vi "Initialize Actor.vi"(7 "Host Name":string, 8 "error in (no error)":errorcluster, 9 "Actor Name":string, 10 "Message Broker Interface":refnum<class "Message Broker Interface.lvclass">, 11 "WS Server in":refnum<class "WS Server.lvclass">) -> (0 "error out":errorcluster, 3 "WS Server out":refnum<class "WS Server.lvclass">)   [LabVIEW 2016, in "WebSocket Networking.lvlib" / "WS Server.lvclass"]
doc: "--\nCopyright © 2017 Composed SystemsI All rights reserved.\n\nAuthor: Jon McBee <jon.mcbee@composed.io>\n\nThis library is provided \"AS IS\" ,WITHOUT WARRANTIES OR\nCONDITIONS OF ANY KIND, either express or implied.\n\nComposed Systems -- composed.io\n\nStream 0.0.1.1\nJon McBee - Composed Systems\nCopyright (c) 2017, Composed Systems"
uses:
  <userlib>/Common Components/WebSocket Networking/WS Server/WS Server.lvclass
  <userlib>/Composed Systems/Stream/Mediator/Classes/Message Broker Interface/Message Broker Interface.lvclass
  <userlib>/Common Components/WebSocket Networking/WS Server/WS Server.lvclass/WS Server.ctl
  <userlib>/Composed Systems/Stream/Mediator/Classes/Websocket Server Actor/Websocket Server/Websocket Server.lvclass
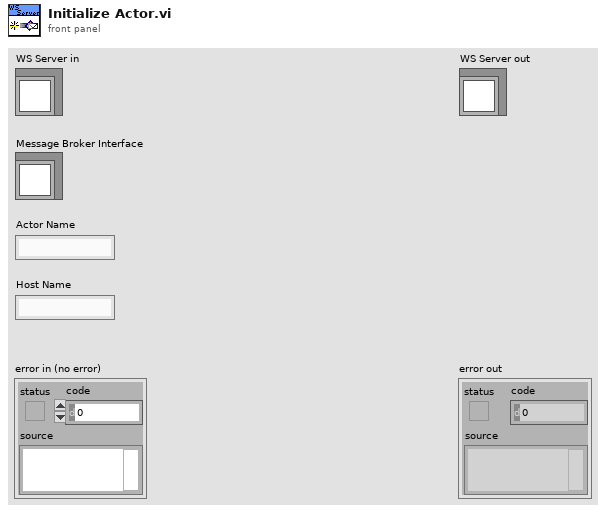
[diagram p1: front panel]
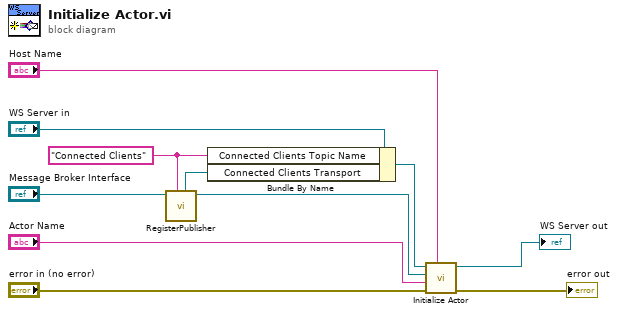
[diagram p0: block diagram]
diagram:
  w1 = "Connected Clients" ("Topic Name")
  n1 = call-dynamic "RegisterPublisher.vi"("Topic Name"=w1, "Message Broker Interface in"="Message Broker Interface") -> ("Message Broker Interface out"=w2:refnum<class "Message Broker Interface.lvclass">, "Transport"=w4:refnum<class "Message Transport Queue.lvclass">)  [unwired: 5 in, 3 out]
  n2 = Bundle By Name(cluster="WS Server in", "Connected Clients Topic Name"=w1, "Connected Clients Transport"=w4) -> (w5:refnum<class "WS Server.lvclass">)
  n3 = call-parent "Initialize Actor.vi"("Host Name"="Host Name", "error in (no error)"="error in (no error)", "Actor Name"="Actor Name", "Message Broker Interface"=w2, "Mediated Asynchronous Actor in"=w5) -> ("error out"=→"error out":errorcluster, "Mediated Asynchronous Actor out"=→"WS Server out":refnum<class "WS Server.lvclass">)  [unwired: 5 in]
